vi "Set Run Control.vi"(8 "error in (no error)":errorcluster, 10 "Run Control":T1, 11 "DPO4104 in":refnum<class "DPO4104.lvclass">) -> (0 "error out":errorcluster, 3 "DPO4104 out":refnum<class "DPO4104.lvclass">)   [LabVIEW 2018, in "DPO4104.lvlib" / "DPO4104.lvclass"]
doc: "This Override method is used to set the Oscope instrument running mode. The 'Run Control' control has 3 modes of operation: 0-Run (or continuous), 1 - Single, 2 - Stop."
uses:
  DPO4104.lvclass
  PPLs/Oscilloscope/Parent/Oscilloscope.lvlibp/Custom Controls/Run Control.ctl
  PPLs/Oscilloscope/Parent/Oscilloscope.lvlibp/Oscilloscope.lvclass
  C:/Projects/LabVIEW/PPLs/Oscilloscope/Parent/Oscilloscope.lvlibp/Oscilloscope.lvclass
  PPLs/Oscilloscope/Parent/Oscilloscope.lvlibp
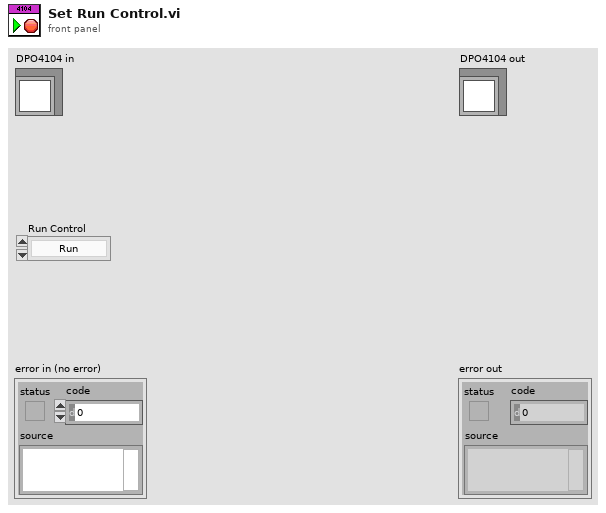
[diagram p1: front panel]
types:
  T1 = typedef "Oscilloscope.lvlibp/Run Control.ctl" = enum16{"Run", "Single", "Stop"}
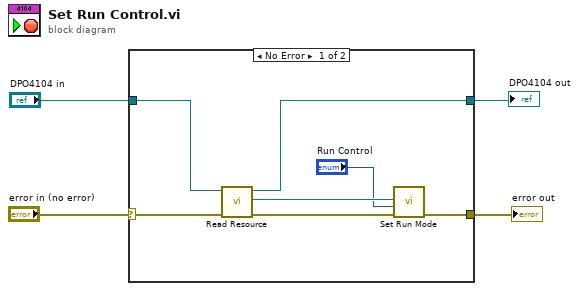
[diagram p0: block diagram]
diagram:
  n1 = case shown="No Error" "error in (no error)" {
    selector: "error in (no error)" -> [w11 w13]
    tunnel: [w6 w13] -> w3
    tunnel: [w9 w12] -> w1
    tunnel: "DPO4104 in" -> [w10 w12]
    frame No Error {
      n2 = call "Read Resource.vi"("error in (no error)"=w11, "Oscilloscope in"=w10) -> ("error out"=w7:errorcluster, "Resource"=w8:refnum<visa-resource-name>, "Oscilloscope out"=w9:refnum<class "DPO4104.lvclass">)  [unwired: 7 in]
      n3 = call "Set Run Mode.vi"("error in (no error)"=w7, "Run Control"="Run Control", "VISA resource name"=w8) -> ("error out"=w6:errorcluster)  [unwired: 7 in, 1 out]
    }
    frame Error {
    }
  }
  "error out" <- w3
  "DPO4104 out" <- w1
